vi "Untitled 5.vi"() -> ()   [LabVIEW 2018]
uses:
  <vilib>/Analysis/coordinate.llb/Euler Rotation Order.ctl
  <vilib>/Analysis/baseanly.llb/Real Inverse Matrix.vi
  <vilib>/imath/engines/lvmath2/RunTimeEngine/NodeEndStatement/NIMS_NodeEndStatement_Output.vi
  <instcachedir>/0/NIMS_NodeEndStatement_Output_53EC0D466D134D7ABD903AC30B43404B.lvgen/NIMS_NodeEndStatement_Output_53EC0D466D134D7ABD903AC30B43404B_009.vi
  <vilib>/imath/engines/lvmath2/RunTimeEngine/ErrorHandling/NIMS_Finalize Error.vi
  <instcachedir>/0/NIMS_NodeEndStatement_Output_53EC0D466D134D7ABD903AC30B43404B.lvgen/NIMS_NodeEndStatement_Output_53EC0D466D134D7ABD903AC30B43404B_004.vi
  <vilib>/Analysis/Matrix/Numeric/Conversions/Array To Matrix - RA.vi
  <vilib>/Analysis/Matrix/Numeric/Conversions/Matrix To Array - RM.vi
  <vilib>/imath/engines/lvmath2/RunTimeEngine/IndexRead/NIMS M(S).vi
  <instcachedir>/0/NIMS M(S)_B826C018497E4940AE96BD27B540B6FB.lvgen/NIMS M(S)_B826C018497E4940AE96BD27B540B6FB_000.vi
  <vilib>/imathl/engines/lvmath/Functions/Error Handling/Create Error.vi
  <vilib>/imath/engines/lvmath2/RunTimeEngine/IndexRead/NIMS V(S).vi
  <instcachedir>/0/NIMS V(S)_0488751826AF41519A22953C041130DC.lvgen/NIMS V(S)_0488751826AF41519A22953C041130DC_000.vi
  <vilib>/imath/engines/lvmath2/RunTimeEngine/BuiltInFunctions/cross/NIMS_cross(GV,GV).vi
  <instcachedir>/0/NIMS_cross(GV,GV)_8E551EB9DC304C30866B49598818C259.lvgen/NIMS_cross(GV,GV)_8E551EB9DC304C30866B49598818C259_000.vi
  <vilib>/imath/engines/lvmath2/RunTimeEngine/BuiltInFunctions/double/NIMS_double.vi
  <instcachedir>/0/NIMS_double_34E32F64C2B04A25A042F4CA881A0A41.lvgen/NIMS_double_34E32F64C2B04A25A042F4CA881A0A41_002.vi
  <instcachedir>/0/NIMS_NodeEndStatement_Output_53EC0D466D134D7ABD903AC30B43404B.lvgen/NIMS_NodeEndStatement_Output_53EC0D466D134D7ABD903AC30B43404B_005.vi
  <vilib>/imath/engines/lvmath2/RunTimeEngine/Managers/WorkSpace/UID Generator.vi
  <vilib>/imath/engines/lvmath2/RunTimeEngine/RunTimeType/NIMS_RunTimeType_From StrictType (excl LVString).vi
  <instcachedir>/0/NIMS_RunTimeType_From StrictType (excl LVString)_E7E34A65C99947108168652BAD14964D.lvgen/NIMS_RunTimeType_From StrictType (excl LVString)_E7E34A65C99947108168652BAD14964D_000.vi
  <vilib>/imath/engines/lvmath2/RunTimeEngine/LocalVariableDefStatement/MC_LocalVariableDefStatement_Display.vi
  <vilib>/imath/engines/lvmath2/RunTimeEngine/ArithmeticOperatorToken/NIMS_ArithmeticOperator_multmx(M,CV).vi
  <instcachedir>/0/NIMS_ArithmeticOperator_multmx(M,CV)_2F1CD6A2FE4F4213A4AD1C901C2750F5.lvgen/NIMS_ArithmeticOperator_multmx(M,CV)_2F1CD6A2FE4F4213A4AD1C901C2750F5_000.vi
  <vilib>/imath/engines/lvmath2/RunTimeEngine/BuiltInFunctions/cross/NIMS_cross(GM,GM,I32).vi
  <instcachedir>/0/NIMS_cross(GM,GM,I32)_0F6D45CF7D834A0BB6695B819A7F63BC.lvgen/NIMS_cross(GM,GM,I32)_0F6D45CF7D834A0BB6695B819A7F63BC_000.vi
  <vilib>/imath/engines/lvmath2/RunTimeEngine/ArithmeticOperatorToken/NIMS_ArithmeticOperator_plus.vi
  <instcachedir>/0/NIMS_ArithmeticOperator_plus_DE670E32103C4C10ADF2A97367172B30.lvgen/NIMS_ArithmeticOperator_plus_DE670E32103C4C10ADF2A97367172B30_003.vi
  <vilib>/imath/engines/lvmath2/RunTimeEngine/ArithmeticOperatorToken/NIMS_ArithmeticOperator_multmx.vi
  <instcachedir>/0/NIMS_ArithmeticOperator_multmx_622CA76F9646436AB036D42A9A1CE0E6.lvgen/NIMS_ArithmeticOperator_multmx_622CA76F9646436AB036D42A9A1CE0E6_004.vi
  <vilib>/imath/engines/lvmath2/RunTimeEngine/ErrorHandling/NIMS_Create Error From Enums.vi
  <vilib>/imath/engines/lvmath2/RunTimeEngine/ArithmeticOperatorToken/NIMS_ArithmeticOperator_multmx-internal.vi
  <instcachedir>/0/NIMS_ArithmeticOperator_multmx-internal_16A6E1DA326644AB974D30232E729C42.lvgen/NIMS_ArithmeticOperator_multmx-internal_16A6E1DA326644AB974D30232E729C42_004.vi
  <vilib>/imath/engines/lvmath2/RunTimeEngine/NodeEndStatement/NIMS_NodeEndStatement_Get Vector.vi
  <instcachedir>/0/NIMS_NodeEndStatement_Get Vector_329D0992E87F49F089135171B7FC9327.lvgen/NIMS_NodeEndStatement_Get Vector_329D0992E87F49F089135171B7FC9327_001.vi
  <vilib>/imath/engines/lvmath/Functions/Error Handling/MergeErrorsWrapper.vi
  <vilib>/imath/engines/lvmath2/RunTimeEngine/Managers/SymbolTable/Clear UID.vi
  <instcachedir>/0/NIMS_NodeEndStatement_Output_53EC0D466D134D7ABD903AC30B43404B.lvgen/NIMS_NodeEndStatement_Output_53EC0D466D134D7ABD903AC30B43404B_003.vi
  <vilib>/Analysis/NI_AALPro.lvlib
  <vilib>/Analysis/Matrix/NI_Matrix.lvlib
  <vilib>/Analysis/NI_AALBase.lvlib
  <vilib>/imath/engines/lvmath2/RunTimeEngine/Managers/SymbolTable/NIMS_WorkSpace.lvlib
panel:
  out "Yaw":dbl(graph)
  out "Pitch":dbl(graph)
  out "Roll":dbl(graph)
  out "W_new":dbl[](array[numeric])
  out "T":dbl[](array[numeric])
  out "Attitude":cluster{"phi":dbl, "theta":dbl, "psi":dbl}
  in  "Mass (kg)":dbl
  in  "MOI(kg*m^2)":dbl[][](array[numeric])
  in  "COG(m)":dbl[](array[numeric])
  in  "Simulation Time(sec)":dbl
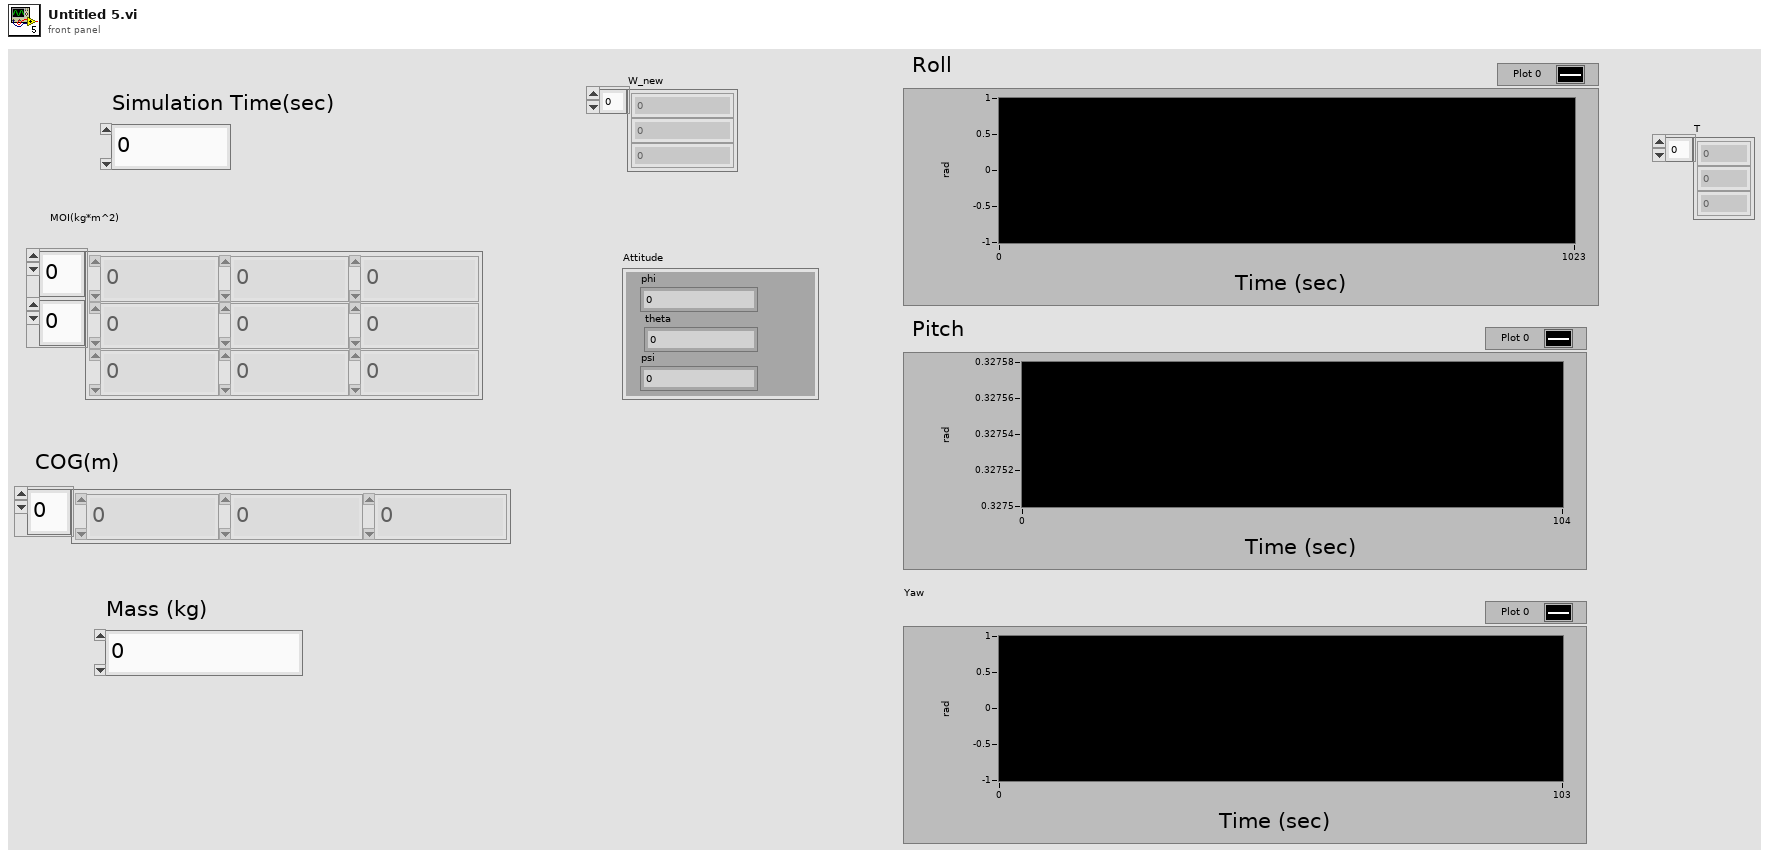
[diagram p1: front panel]
types:
  T1 = typedef "NI_Matrix.lvlib/RealMatrix.ctl" = dbl[][]
  T2 = typedef "NI_AALPro.lvlib/Euler Rotation Order.ctl" = u16
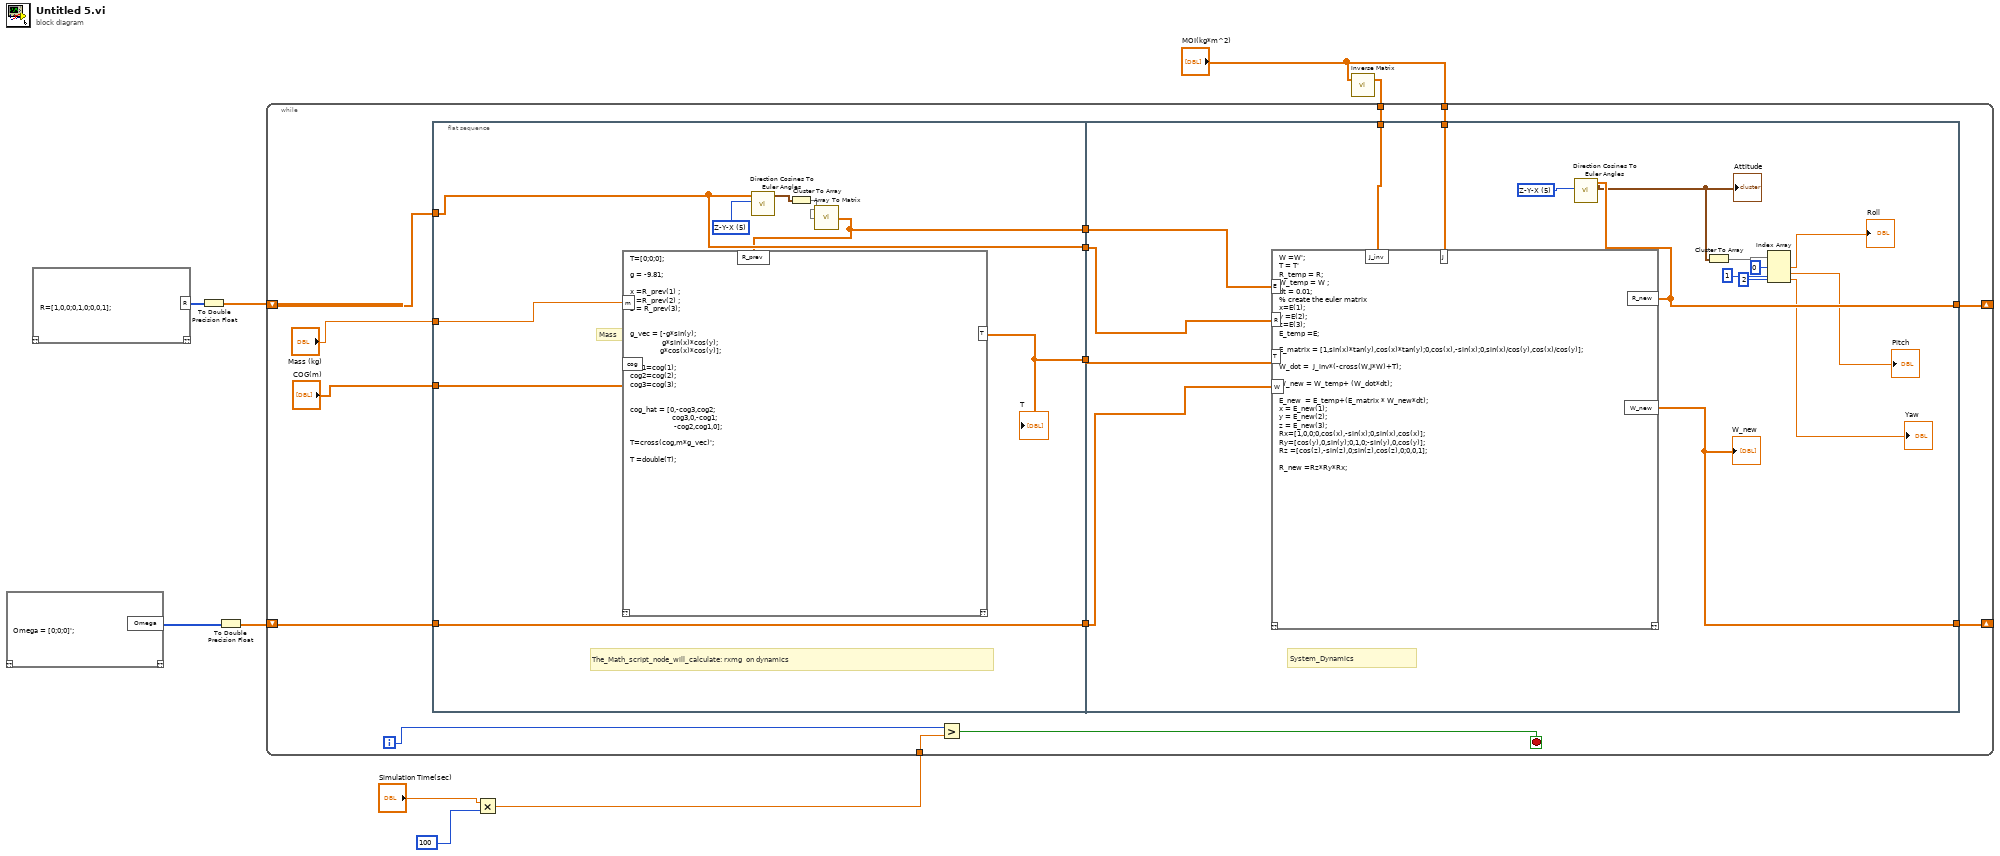
[diagram p0: block diagram]
diagram:
  n1 = mathscript code="Omega = [0;0;0]';"() -> ("Omega"=w6:i32[])  [unwired: 1 in, 1 out]
  n2 = mathscript code="R=[1,0,0;0,1,0;0,0,1];"() -> ("R"=w9:i32[][])  [unwired: 1 in, 1 out]
  n3 = To Double Precision Float(number=w9) -> (double precision float=w8:dbl[][])
  n4 = To Double Precision Float(number=w6) -> (double precision float=w7:dbl[])
  n5 = Multiply(x="Simulation Time(sec)", y=100) -> (x*y=w3:dbl)
  n6 = call-poly <vilib>:"Inverse Matrix.vi"("Input Matrix"="MOI(kg*m^2)") -> ("Inverse Matrix"=w1:T1)  [unwired: 1 in, 1 out]
  n7 = while {
    shift-right: [w23] -> _
    shift-left: w8 -> [w24]
    shift-right: [w13] -> _
    shift-left: w7 -> [w21]
    tunnel: w3 -> [w18]
    tunnel: "MOI(kg*m^2)" -> [w12]
    tunnel: w1 -> [w11]
    i -> [w19]
    stop <- w17 stop-if-true
    n8 = flat-sequence {
      tunnel: w24 -> [w28]
      tunnel: "Mass (kg)" -> [w30]
      tunnel: "COG(m)" -> [w29]
      tunnel: [w27] -> w22
      tunnel: w21 -> [w27]
      tunnel: [w28] -> w20
      tunnel: [w26] -> w14
      tunnel: [w25] -> w10
      tunnel: [w253] -> w23
      tunnel: w22 -> [w258]
      tunnel: w20 -> [w260]
      tunnel: w14 -> [w259]
      tunnel: [w257] -> w13
      tunnel: w12 -> [w256]
      tunnel: w11 -> [w255]
      tunnel: w10 -> [w254]
      frame #0 {
        w31 = T2 5 items=["X-Y-Z", "X-Z-Y", "Y-X-Z", "Y-Z-X", "Z-X-Y", "Z-Y-X", "X-Y-X", "X-Z-X", "Y-X-Y", "Y-Z-Y", "Z-X-Z", "Z-Y-Z"] ("rotation order")
        # "Mass"
        # "The_Math_script_node_will_calculate: rxmg  on dynamics"
        n9 = call <vilib>:"Direction Cosines To Euler Angles.vi"("rotation order"=w31, "Direction Cosines"=w28) -> ("Euler Angles"=w33:cluster{"phi":dbl, "theta":dbl, "psi":dbl})  [unwired: 8 in, 1 out]
        n10 = Cluster To Array(cluster=w33) -> (array=w32:dbl[])
        n11 = call-poly <vilib>:"Array To Matrix.vi"("Real 1D Array"=w32) -> ("Real Matrix (Column Vector)"=w25:T1)
        n12 = mathscript code="T=[0;0;0];\n\ng = -9.81;\n\nx =R_prev(1) ;\ny =R_prev(2) ;\nz = R_prev(3);\n\n\ng_vec = [-g*sin(y);\n                g*sin(x)*cos(y);\n               g*cos(x)*cos(y)];\n\ncog1=cog(1);\ncog2=cog(2);\ncog3=cog(3);\n\n\ncog_hat = [0,-cog3,cog2;\n                     cog3,0,-cog1;\n                      -cog2,cog1,0];\n\nT=cross(cog,m*g_vec)';\n\nT =double(T);"("m"=w30, "cog"=w29, "R_prev"=w25) -> ("T"=w26:dbl[])  [unwired: 1 in, 1 out]
        "T" <- w26
      }
      frame #1 {
        w261 = T2 5 items=["X-Y-Z", "X-Z-Y", "Y-X-Z", "Y-Z-X", "Z-X-Y", "Z-Y-X", "X-Y-X", "X-Z-X", "Y-X-Y", "Y-Z-Y", "Z-X-Z", "Z-Y-Z"] ("rotation order")
        # "System_Dynamics"
        n13 = mathscript code="W =W';\nT = T'\nR_temp = R;\nW_temp = W ;\ndt = 0.01;\n% create the euler matrix\nx=E(1);\ny =E(2);\nz=E(3);\nE_temp =E;\n\nE_matrix = [1,sin(x)*tan(y),cos(x)*tan(y);0,cos(x),-sin(x);0,sin(x)/cos(y),cos(x)/cos(y)];\n\nW_dot =  J_inv*(-cross(W,J*W)+T);\n\nW_new = W_temp+ (W_dot*dt);\n\nE_new  = E_temp+(E_matrix * W_new*dt);\nx = E_new(1);\ny = E_new(2);\nz = E_new(3);\nRx=[1,0,0;0,cos(x),-sin(x);0,sin(x),cos(x)];\nRy=[cos(y),0,sin(y);0,1,0;-sin(y),0,cos(y)];\nRz =[cos(z),-sin(z),0;sin(z),cos(z),0;0,0,1];\n\nR_new =Rz*Ry*Rx;"("J"=w256, "R"=w260, "T"=w259, "W"=w258, "J_inv"=w255, "E"=w254) -> ("R_new"=w253:cdb[][], "W_new"=w257:dbl[])  [unwired: 1 in, 1 out]
        "W_new" <- w257
        n14 = call <vilib>:"Direction Cosines To Euler Angles.vi"("rotation order"=w261, "Direction Cosines"=w253) -> ("Euler Angles"=w252:cluster{"phi":dbl, "theta":dbl, "psi":dbl})  [unwired: 8 in, 1 out]
        "Attitude" <- w252
        n15 = Cluster To Array(cluster=w252) -> (array=w251:dbl[])
        n16 = Index Array(array=w251, index #1=0 ("index"), index #2=1 ("index"), index #3=2 ("index")) -> (element #1=→"Roll":dbl, element #2=→"Pitch":dbl, element #3=→"Yaw":dbl)
      }
    }
    n17 = Greater?(x=w19, y=w18) -> (0:w17:bool)
  }
